vi "Read Excel Data.vi"(8 "error in (no error)":errorcluster caption="错误输入（无错误）") -> (0 "error out":errorcluster caption="错误输出", 1 "Type":string[](array[string]), 2 "IP Address":string[](array[string]), 3 "Device Name":string[](array[string]))   [LabVIEW 2018]
uses:
  <vilib>/Utility/NIReport.llb/Report Type.ctl
  <vilib>/addons/_office/excel.llb/Excel Get Data ([str]).vi
  <vilib>/Utility/NIReport.llb/NI_report.lvclass
  <vilib>/Utility/NIReport.llb/Excel/NI_Excel.lvclass
  <vilib>/Utility/NIReport.llb/NI_ReportGenerationCore.lvlib
  <vilib>/addons/_office/NI_ReportGenerationToolkit.lvlib
panel:
  out "表格控件":string[][](table)
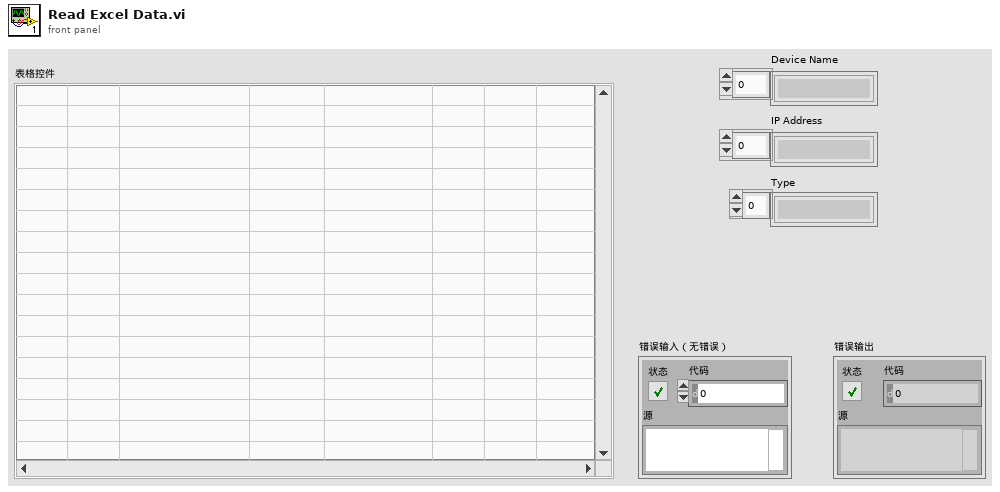
[diagram p1: front panel]
types:
  T1 = enum16{"maximized", "minimized", "normal", "no change"}
  T2 = typedef "NI_ReportGenerationCore.lvlib/Report Type.ctl" = enum16{"HTML", "Word", "Excel"}
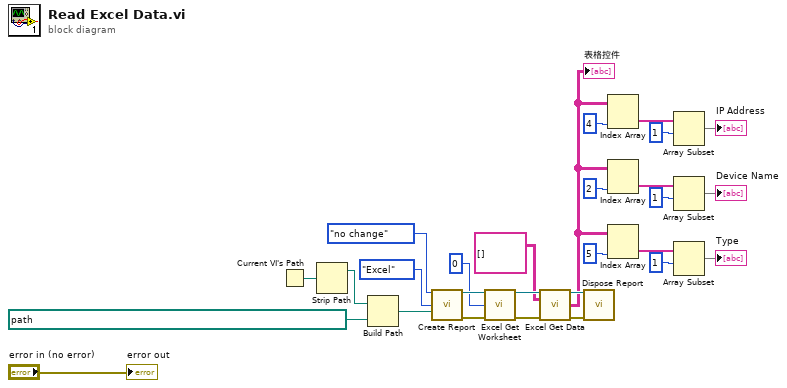
[diagram p0: block diagram]
diagram:
  n1 = Current VI's Path() -> (path=w5:path)
  n2 = Strip Path(path=w5) -> (stripped path=w4:path)  [unwired: 1 out]
  n3 = Build Path(base path=w4, name or relative path=path "../Document/7.交直流配电板及其配电开关IP地址需求表.xlsx" ("template (empty)")) -> (appended path=w3:path)
  n4 = call <vilib>:"Create Report.vi"("window state (normal)"=T1."no change", "report type"=Report_Type."Excel", "template (empty)"=w3) -> ("report out"=w15:refnum<class "NI_report.lvclass">, "error out"=w13:errorcluster)  [unwired: 11 in]
  n5 = call <vilib>:"Excel Get Worksheet.vi"("report in"=w15, "worksheet index (0)"=0, "error in (no error)"=w13) -> ("report out"=w10:refnum<class "NI_report.lvclass">, "error out"=w7:errorcluster)  [unwired: 11 in]
  n6 = call-poly <vilib>:"Excel Get Data.vi"("report in"=w10, "data type"=string[][] [], "error in (no error)"=w7) -> ("report out"=w9:refnum<class "NI_report.lvclass">, "data"=w1:string[][], "error out"=w6:errorcluster)  [unwired: 10 in]
  "表格控件" <- w1
  n7 = call-dynamic "Dispose Report.vi"("report in"=w9, "error in (no error)"=w6) -> ()  [unwired: 13 in, 1 out]
  n8 = Index Array(array=w1, index (col)=4 ("禁用的索引 (列)")) -> (element=w26:string[])  [unwired: 1 in]
  n9 = Index Array(array=w1, index (col)=2 ("禁用的索引 (列)")) -> (element=w23:string[])  [unwired: 1 in]
  n10 = Index Array(array=w1, index (col)=5 ("禁用的索引 (列)")) -> (element=w19:string[])  [unwired: 1 in]
  n11 = Array Subset(array=w26, index=1 ("索引")) -> (→"IP Address":string[])  [unwired: 1 in]
  n12 = Array Subset(array=w23, index=1 ("索引")) -> (→"Device Name":string[])  [unwired: 1 in]
  n13 = Array Subset(array=w19, index=1 ("索引")) -> (→"Type":string[])  [unwired: 1 in]
  "error out" <- "error in (no error)"
